vi "areaSettiingDlg.vi"(8 "error in (no error)":errorcluster caption="错误输入（无错误）", 11 "区域管理":T1 {"电极排列方式" items=["等间隔十字排列", "等间隔一字排列", "等间隔错位排列"]}) -> (0 "error out":errorcluster caption="错误输出（无错误）", 3 "区域管理 out":T1)   [LabVIEW 2014, in "SettingD.lvlib"]
uses:
  SettingD.llb/SettingD.lvlib
  DataBase/DataBase.lvlib
panel:
  in  "OK":bool
  in  "取消按钮":bool
  in  "确定按钮":bool
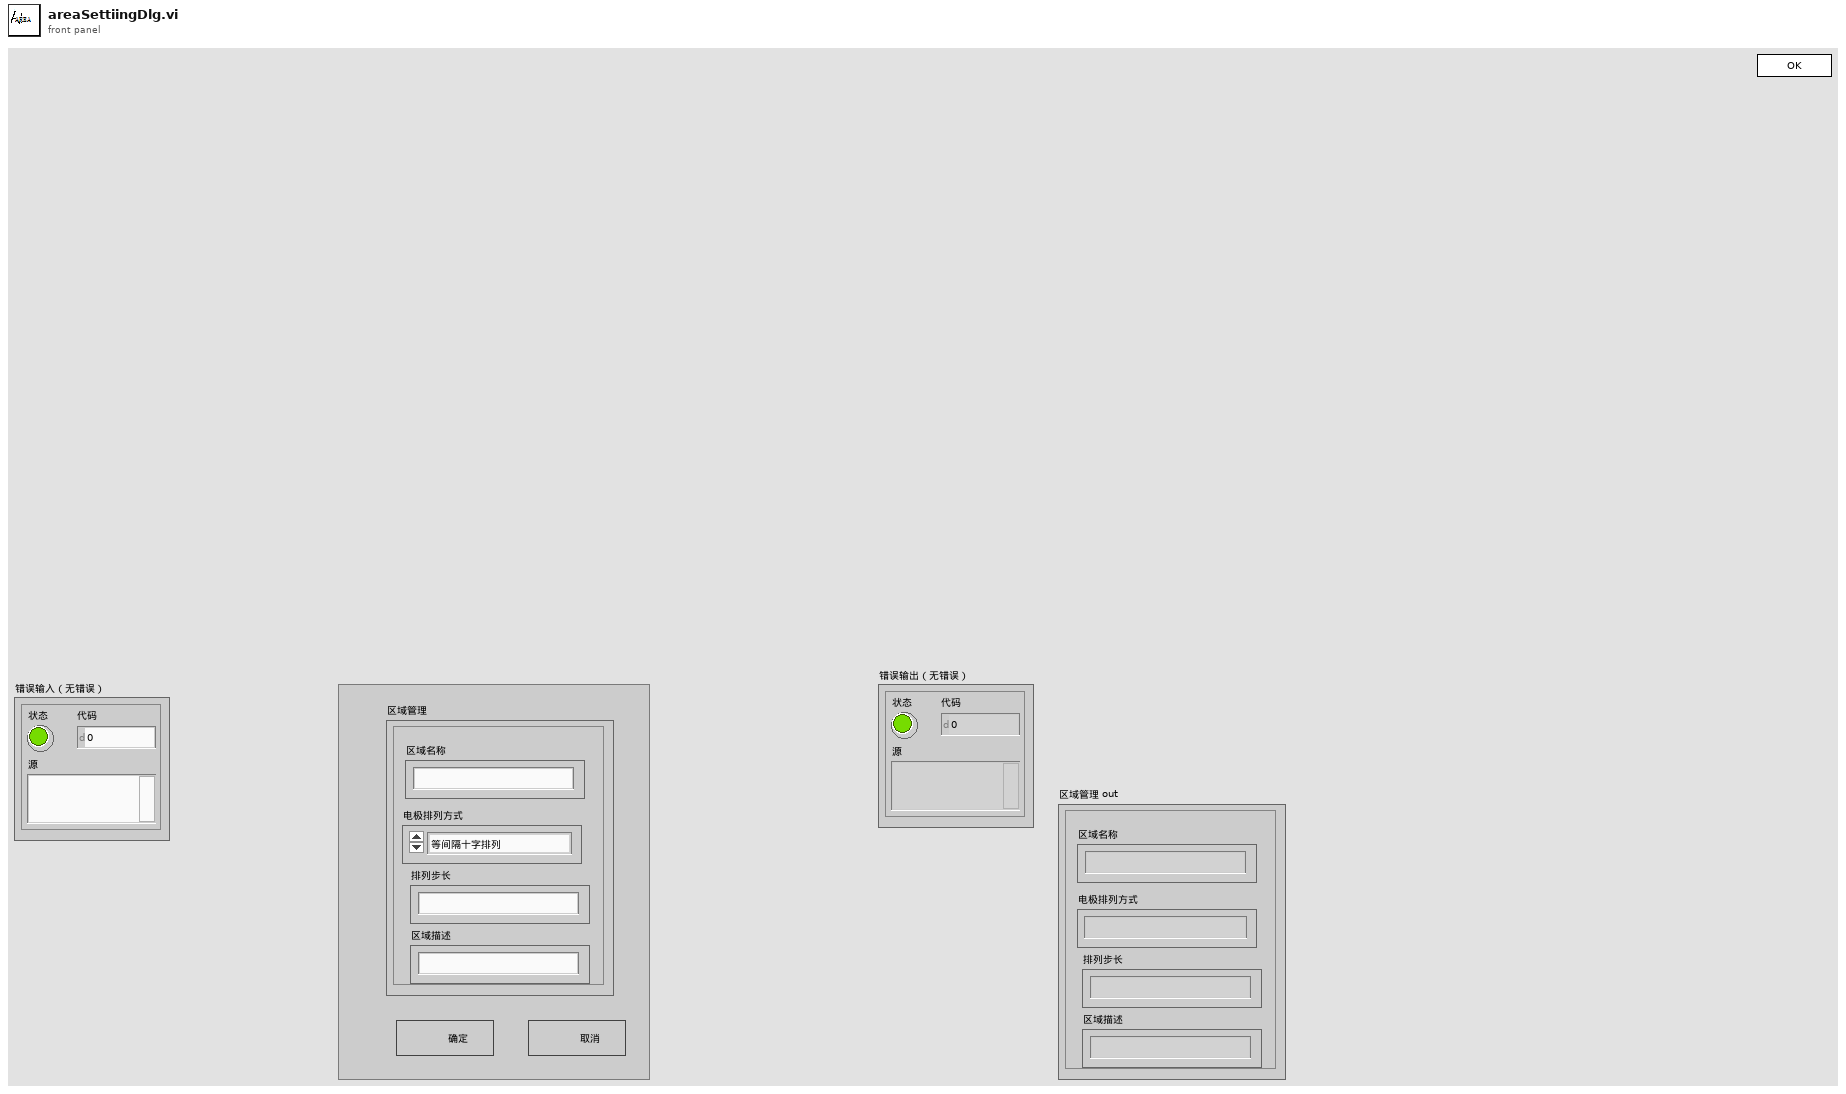
[diagram p1: front panel]
types:
  T1 = cluster{"区域名称":string, "电极排列方式":u16, "排列步长":string, "区域描述":string}
  T2 = enum32{"invalid app kind", "Development System", "Run Time System", "Student Edition", "Embedded LabVIEW", "Evaluation", "Custom"}
  T3 = enum32{"Invalid", "Standard", "Closed", "Hidden", "Minimized", "Maximized"}
  T4 = cluster{i32, "区域名称":string, string, "排列步长":string, "区域描述":string}
  T5 = cluster{"Core":cluster{"Current VI Reference":refnum<vi>, "Close Panel on Exit?":bool}, "Your Boolean data":bool, "Your string data":string}
  T6 = cluster{"Current VI Reference":refnum<vi>, "Close Panel on Exit?":bool}
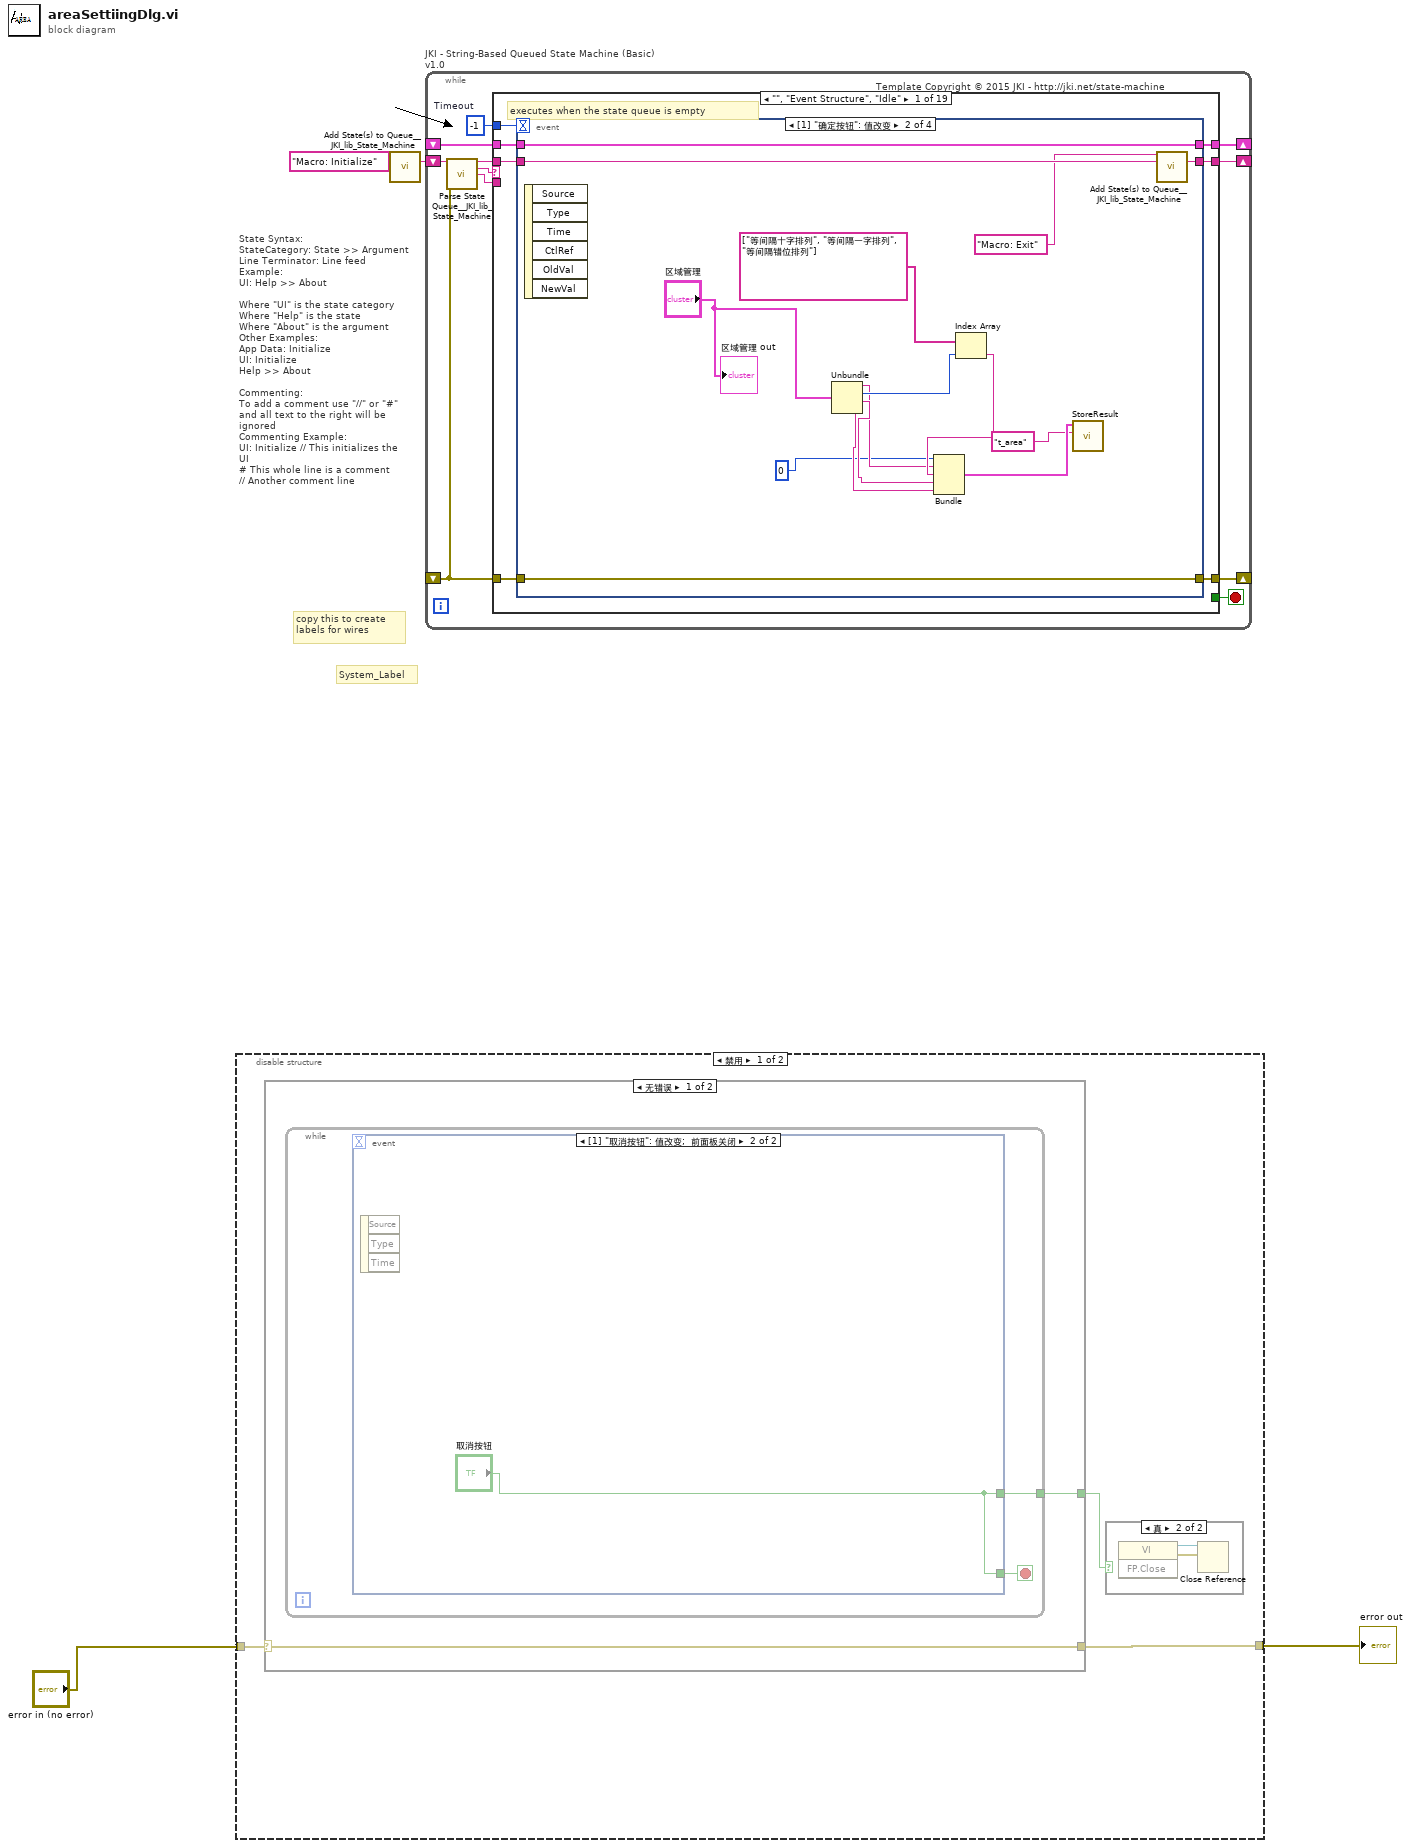
[diagram p0: block diagram]
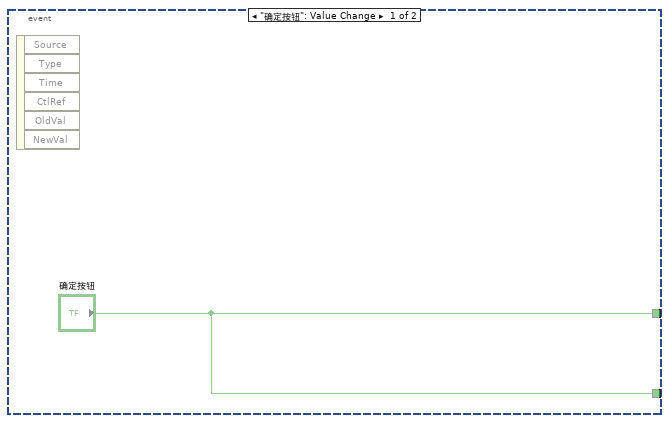
[diagram p2: hidden frame]
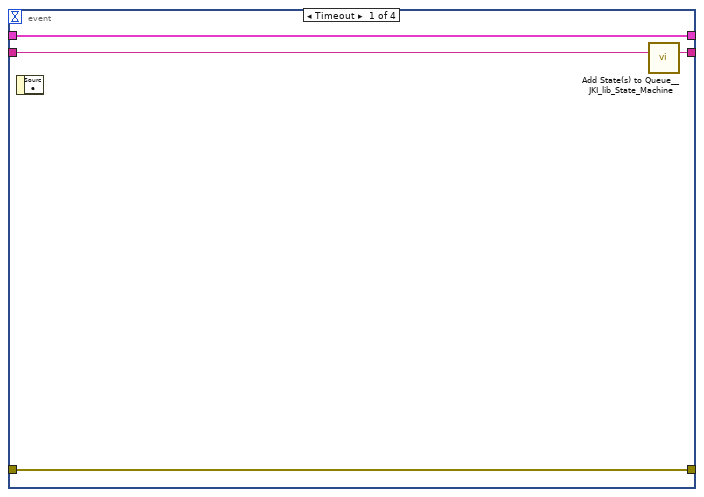
[diagram p6: hidden frame]
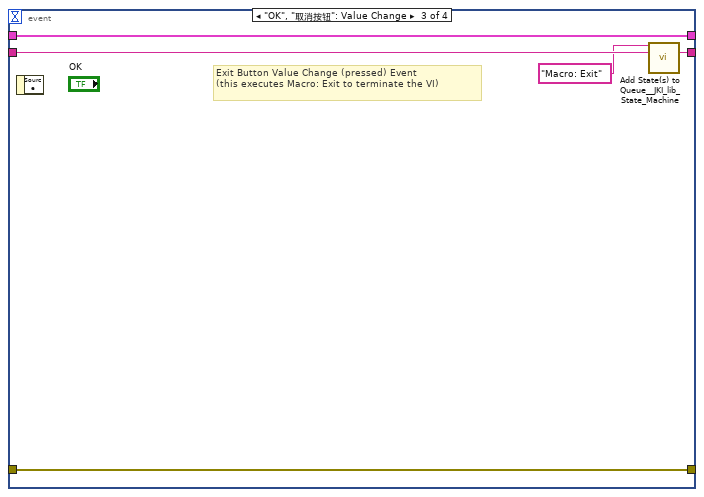
[diagram p7: hidden frame]
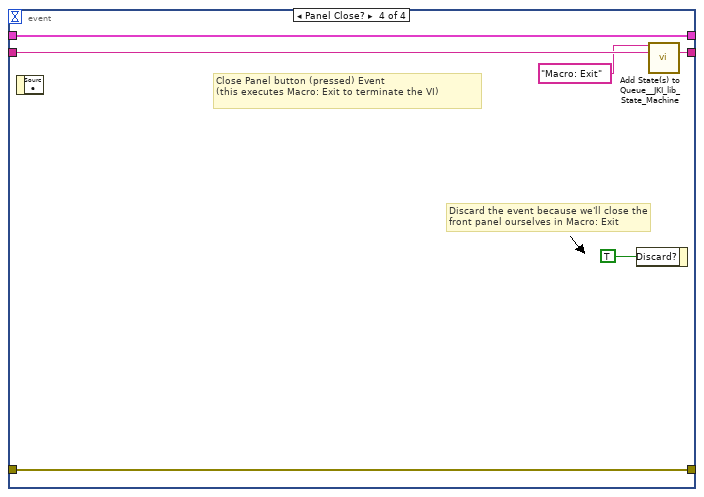
[diagram p8: hidden frame]
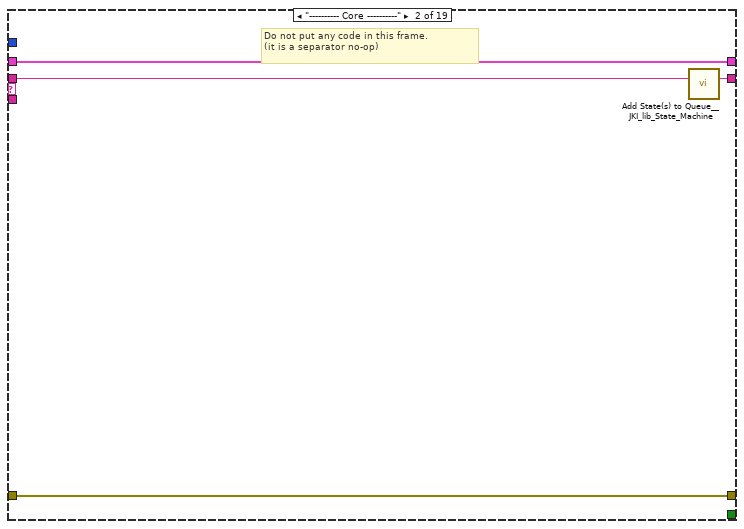
[diagram p9: hidden frame]
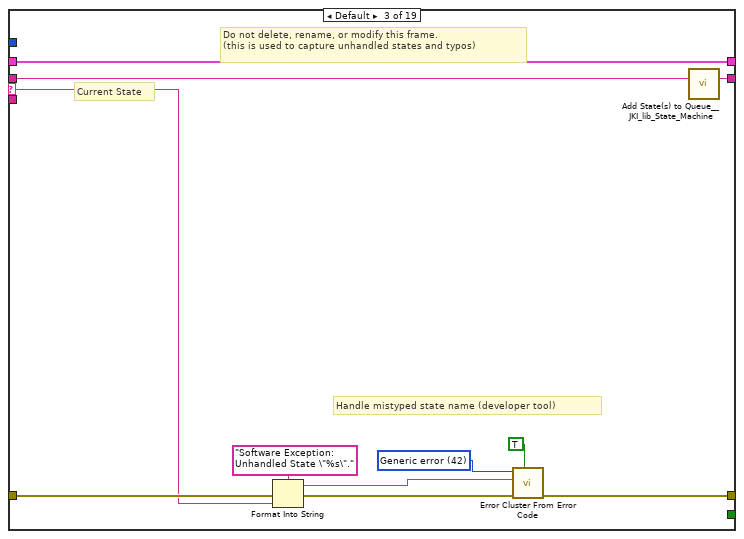
[diagram p10: hidden frame]
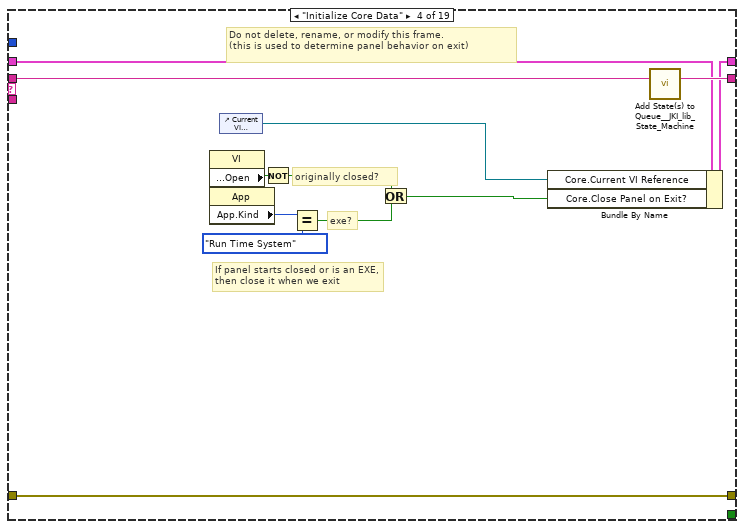
[diagram p11: hidden frame]
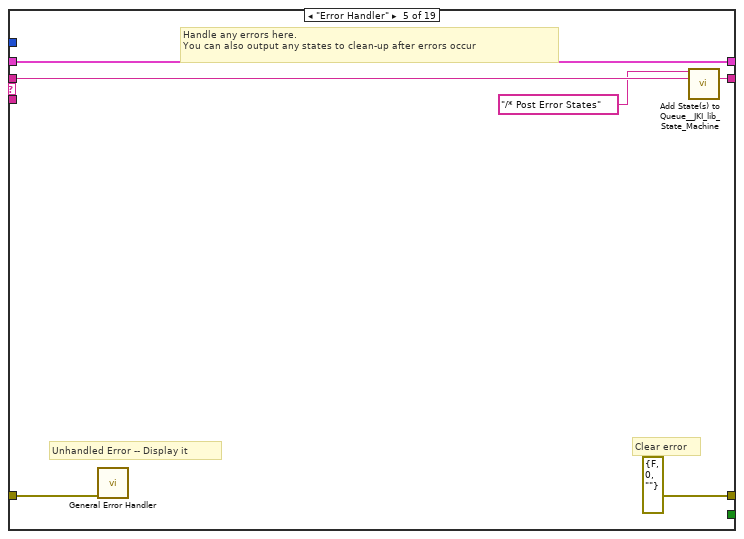
[diagram p12: hidden frame]
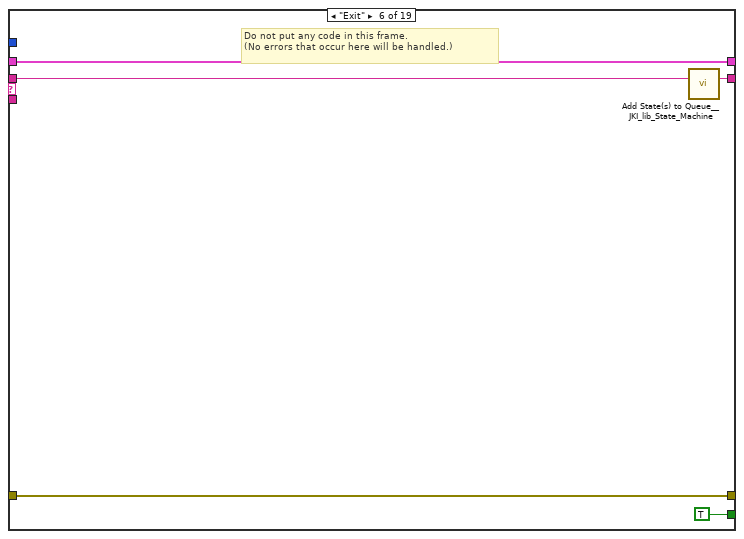
[diagram p13: hidden frame]
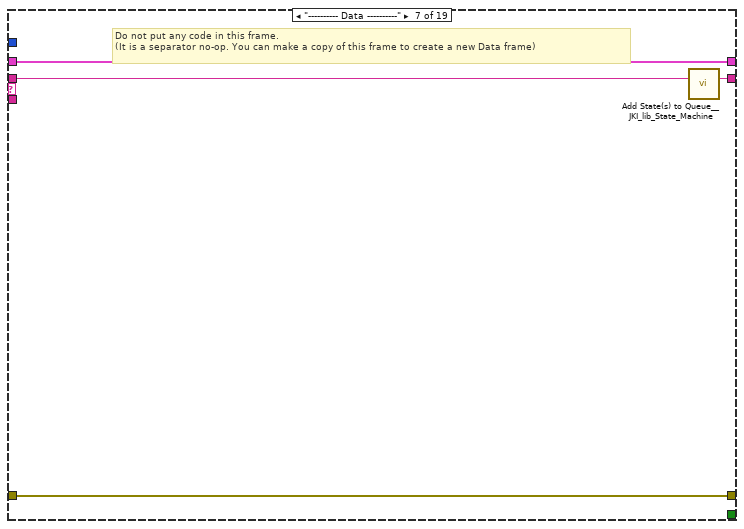
[diagram p14: hidden frame]
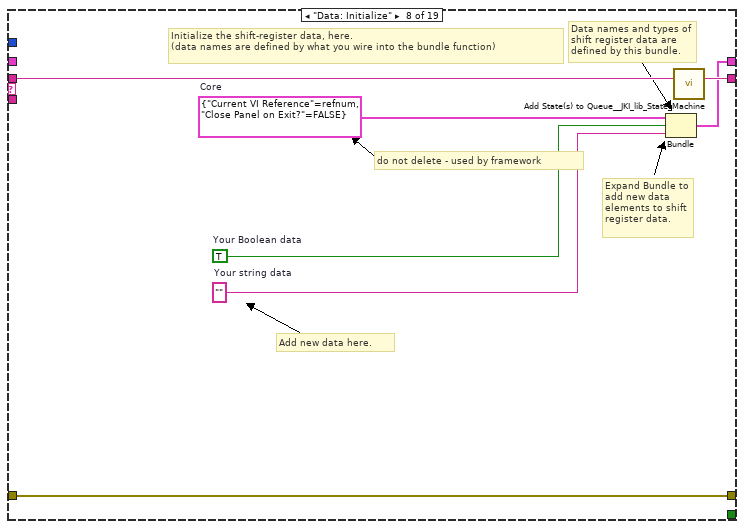
[diagram p15: hidden frame]
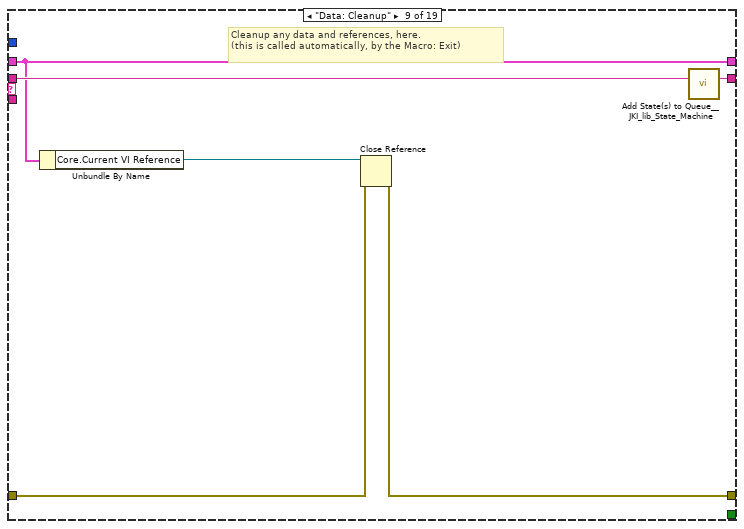
[diagram p16: hidden frame]
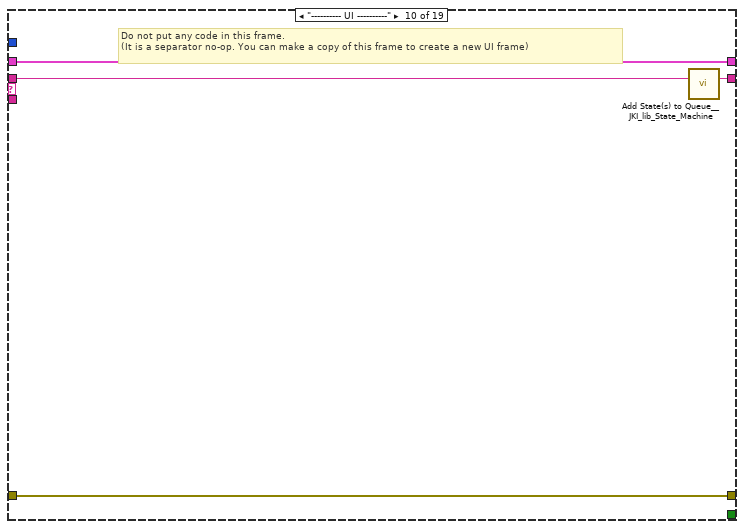
[diagram p17: hidden frame]
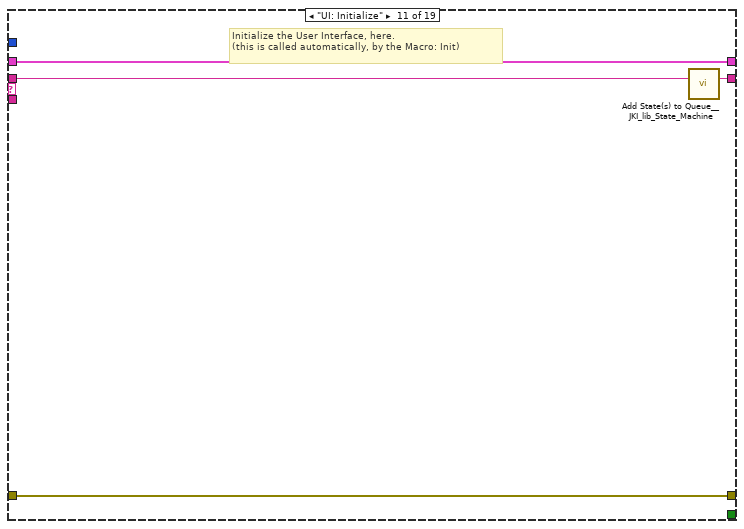
[diagram p18: hidden frame]
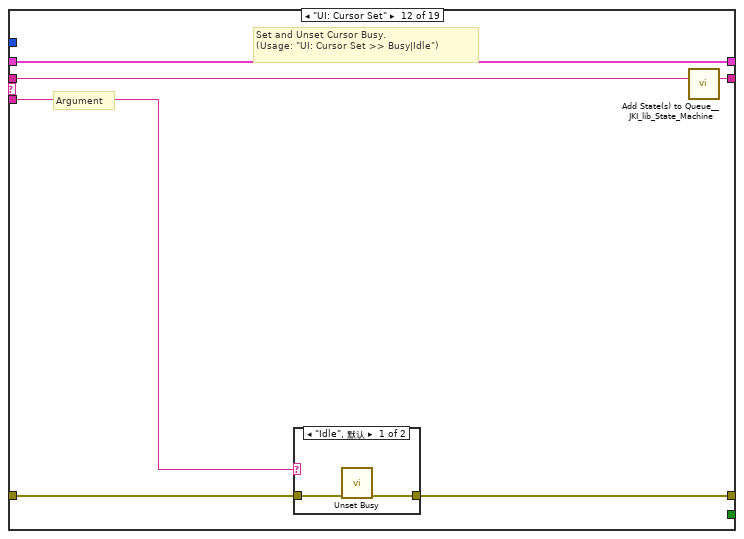
[diagram p19: hidden frame]
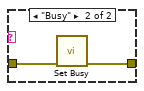
[diagram p20: hidden frame]
diagram:
  # "State Syntax:\nStateCategory: State >> Argument\nLine Terminator: Line feed\nExample:\nUI: Help >> About\n\nWhere \"UI\" is the state category\nWhere \"Help\" is the state\nWhere \"About\" is the argument\nOther Examples:\nApp Data: Initialize\nUI: Initialize\nHelp >> About\n\nCommenting:\nTo add a comment use \"//\" or \"#\" and all text to the right will be ignored\nCommenting Example:\nUI: Initialize // This initializes the UI\n# This whole line is a comment\n// Another comment line"
  # "copy this to create labels for wires"
  # "System_Label"
  n1 = disable-structure shown="禁用" {
    disable-tunnel: "error in (no error)" -> [w7 _]
    disable-tunnel: [w6 _] -> w3
    frame Disabled {
      n2 = case shown="无错误" w7 {
        selector: w7 -> [w9 w14]
        tunnel: [w9 w14] -> w6
        tunnel: [w8 _] -> w5
        frame No Error {
          n3 = while {
            tunnel: [w11] -> w8
            stop <- w10 stop-if-true
            n4 = event shown="[1] \"取消按钮\": 值改变;  前面板关闭" {
              selector: _ -> [_ _]
              dyn-events: _ -> [_ _]
              timeout: _ -> [_ _]
              tunnel: ["确定按钮" "取消按钮"] -> w11
              tunnel: ["确定按钮" "取消按钮"] -> w10
              event "确定按钮": Value Change {
                n5 = event-data() -> ()  [unwired: 1 in, 6 out]
              }
              event "取消按钮": Value Change; Panel Close {
                n6 = event-data() -> ()  [unwired: 1 in, 3 out]
              }
            }
          }
        }
        frame Error {
        }
      }
      n7 = case shown="真" w5 {
        frame False {
        }
        frame True {
          n8 = invoke class="VI" method="FP.Close"() -> (reference out=w16:refnum<vi>, error out=w15:errorcluster)  [unwired: 3 in, 1 out]
          n9 = Close Reference(reference=w16, error in (no error)=w15) -> ()  [unwired: 1 out]
        }
      }
    }
    frame Enabled {
    }
  }
  "error out" <- w3
  n10 = call <vilib>:"Add State(s) to Queue__JKI_lib_State_Machine.vi"("State(s) in (\"\")"="Macro: Initialize") -> ("States Out"=w2:string)  [unwired: 14 in]
  n11 = while "JKI - String-Based Queued State Machine (Basic) v1.0" {
    shift-right: [w20] -> _
    shift-left: _ -> [w19]
    shift-right: [w23] -> _
    shift-left: _ -> [w17]
    shift-right: [w22] -> _
    shift-left: w2 -> [w24]
    stop <- w21 stop-if-true
    w18 = -1  # Timeout
    # "Template Copyright © 2015 JKI - http://jki.net/state-machine"
    n12 = call <vilib>:"Parse State Queue__JKI_lib_State_Machine.vi"("State Queue"=w24, "Error In (no error)"=w17) -> ("Remaining States"=w26:string, "Current State"=w27:string, "Arguments"=w25:string)  [unwired: 11 in]
    n13 = case shown="\"\", \"Event Structure\", \"Idle\"" w27 {
      selector: w27 -> [_ _ w69 _ _ _ _ _ _ _ _ _ _ _ _ _ _ _ _]
      tunnel: w26 -> [w34 w68 w73 w91 w97 w102 w106 w113 w119 w123 w127 w133 w144 w170 w175 w185 w189 w193 w197]
      tunnel: w25 -> [_ _ _ _ _ _ _ _ _ _ _ w128 w138 _ _ _ _ _ _]
      tunnel: w19 -> [w32 w65 w71 w82 w94 w100 w103 _ w114 w120 w125 w131 w140 w167 w172 w182 w186 w190 w194]
      tunnel: [w31 w66 w75 w88 errorcluster {"status"=FALSE, "code"=0, "source"=""} ("error out") w99 w104 w110 w115 w121 w124 w129 w141 w168 w173 w183 w187 w191 w195] -> w23
      tunnel: w17 -> [w30 w66 w74 w88 w93 w99 w104 w110 w116 w121 w124 w130 w142 w168 w173 w183 w187 w191 w195]
      tunnel: [w33 w67 w72 w90 w96 w101 w105 w112 w118 w122 w126 w132 w143 w169 w174 w184 w188 w192 w196] -> w22
      tunnel: [_ _ _ _ _ TRUE _ _ _ _ _ _ _ _ _ _ _ _ _] -> w21
      tunnel: [w29 w65 w71 w89 w94 w100 w103 w111 w114 w120 w125 w131 w140 w167 w172 w182 w186 w190 w194] -> w20
      tunnel: w18 -> [w28 _ _ _ _ _ _ _ _ _ _ _ _ _ _ _ _ _ _]
      frame "", "Event Structure", "Idle" {
        # "executes when the state queue is empty"
        n14 = event shown="[1] \"确定按钮\": 值改变" {
          selector: _ -> [_ _ _ _]
          dyn-events: _ -> [_ _ _ _]
          timeout: w28 -> [_ _ _ _]
          tunnel: w34 -> [w38 w53 w58 w64]
          tunnel: [w37 w52 w57 w63] -> w33
          tunnel: w32 -> [w35 w50 w55 w61]
          tunnel: [w36 w51 w56 w62] -> w31
          tunnel: w30 -> [w36 w51 w56 w62]
          tunnel: [w35 w50 w55 w61] -> w29
          event Timeout {
            n15 = event-data() -> ()  [unwired: 1 in, 1 out]
            n16 = call <vilib>:"Add State(s) to Queue__JKI_lib_State_Machine.vi"("State(s) in (\"\")"=w38) -> ("States Out"=w37:string)  [unwired: 14 in]
          }
          event "确定按钮": Value Change {
            n17 = event-data() -> ()  [unwired: 1 in, 6 out]
            n18 = Unbundle("区域管理") -> ("区域名称"=w43:string, "电极排列方式"=w47:u16, "排列步长"=w44:string, "区域描述"=w45:string)
            n19 = Index Array(array=string[] ["等间隔十字排列", "等间隔一字排列", "等间隔错位排列"], index=w47) -> (element=w48:string)
            n20 = Bundle(0, "区域名称"=w43, w48, "排列步长"=w44, "区域描述"=w45) -> (w49:T4)  [unwired: 1 in]
            n21 = call "StoreResult.vi"("Table name"="t_area", "区域管理"=w49) -> ()  [unwired: 9 in, 1 out]
            n22 = call <vilib>:"Add State(s) to Queue__JKI_lib_State_Machine.vi"("State(s) in Front (\"\")"="Macro: Exit", "State(s) in (\"\")"=w53) -> ("States Out"=w52:string)  [unwired: 13 in]
            "区域管理 out" <- "区域管理"
          }
          event "OK", "取消按钮": Value Change {
            # "Exit Button Value Change (pressed) Event\n(this executes Macro: Exit to terminate the VI)"
            n23 = event-data() -> ()  [unwired: 1 in, 1 out]
            n24 = call <vilib>:"Add State(s) to Queue__JKI_lib_State_Machine.vi"("State(s) in Front (\"\")"="Macro: Exit", "State(s) in (\"\")"=w58) -> ("States Out"=w57:string)  [unwired: 13 in]
          }
          event Panel Close? {
            # "Discard the event because we'll close the front panel ourselves in Macro: Exit"
            # "Close Panel button (pressed) Event\n(this executes Macro: Exit to terminate the VI)"
            n25 = event-data() -> ()  [unwired: 1 in, 1 out]
            n26 = event-data("Discard?"=TRUE) -> ()  [unwired: 1 in, 1 out]
            n27 = call <vilib>:"Add State(s) to Queue__JKI_lib_State_Machine.vi"("State(s) in Front (\"\")"="Macro: Exit", "State(s) in (\"\")"=w64) -> ("States Out"=w63:string)  [unwired: 13 in]
          }
        }
      }
      frame "---------- Core ----------" {
        # "Do not put any code in this frame.\n(it is a separator no-op)"
        n28 = call <vilib>:"Add State(s) to Queue__JKI_lib_State_Machine.vi"("State(s) in (\"\")"=w68) -> ("States Out"=w67:string)  [unwired: 14 in]
      }
      frame Default {
        w78 = 42 items=["No error", "Argument error", "Memory is full", "Out of zone", "End of file", "File already open", "Generic file I/O error", "File not found", "File permission error", "Disk is full", "Duplicate path", "Too many files open", "System feature not enabled", "Resource file not found", "Cannot add resource", "Resource not found", "Image not found", "Image memory error", "Pen does not exist", "Config type invalid", "Config token not found", "Config parse error", "Config memory error", "Bad external code format", "Bad external code offset", "External code not present", "Null window", "Destroy window error", "Null menu", "Print aborted", "Bad print record", "Print driver error", "Windows error during printing", "Memory error during printing", "Print dialog error", "Generic print error", "Invalid device refnum", "Device not found", "Device parameter error", "Device unit error", "Cannot open device", "Device call aborted", "Generic error", "Cancelled by user", "Object ID too low", "Object ID too high", "Object not in heap", "Unknown heap", "Unknown object (invalid DefProc)", "Unknown object (DefProc not in table)", "Message out of range", "Invalid (null) method", "Unknown message", "Manager call not supported", "Bad address", "Network operation in progress", "Network operation timed out", "Connection is busy", "Network attribute not supported", "Network error", "Address in use", "System out of memory", "Connection aborted", "Connection refused", "Not connected", "Already connected", "Connection closed", "Initialization error (interapplication manager)", "Bad occurrence", "Wait on unbound occurrence handler", "Occurrence queue overflow", "Datalog type conflict", "Unused", "Unrecognized type (interapplication manager)", "Memory corrupt", "Failed to make temporary DLL", "Old CIN version", "Drag socket not found", "Failed to load drop-object", "Failed to register OLE object", "Failed to release OLE object", "Format specifier type mismatch", "Unknown format specifier", "Too few format specifiers", "Too many format specifiers", "Scan failed", "Newer CIN version", "Error converting to variant", "Runtime menu error", "Password tampered", "Variant attribute not found", "Incompatible variant data type", "Event data is not available", "Event Store is not present", "Occurrence is not found", "Event Queue is not created", "Event info is not available", "Refnum passed is NULL", "Error retrieving Class GUID", "Error retrieving CoClass GUID", "Error retrieving TypeLib GUID.", "Bad built application magic bytes.", "Specific driver is different from the specific driver associated with the Logical Name.", "There is no session opened to the class driver.", "Max Error", "MAX - Error with config objects", "MAX - Error loading configuration", "MAX - Group not supported"]
        # "Current State"
        # "Do not delete, rename, or modify this frame.\n(this is used to capture unhandled states and typos)"
        # "Handle mistyped state name (developer tool)"
        n29 = Format Into String(format string="Software Exception: Unhandled State \"%s\"." ("message"), error in=w74, w69) -> (resulting string=w77:string, error out=w76:errorcluster)  [unwired: 1 in]
        n30 = call <vilib>:"Error Cluster From Error Code.vi"("show call chain? (False)"=TRUE, "error in (no error)"=w76, "error message (\"\")"=w77, "error code (0)"=w78) -> ("error out"=w75:errorcluster)  [unwired: 5 in]
        n31 = call <vilib>:"Add State(s) to Queue__JKI_lib_State_Machine.vi"("State(s) in (\"\")"=w73) -> ("States Out"=w72:string)  [unwired: 14 in]
      }
      frame "Initialize Core Data" {
        # "Do not delete, rename, or modify this frame.\n(this is used to determine panel behavior on exit)"
        # "originally closed?"
        # "exe?"
        # "If panel starts closed or is an EXE, then close it when we exit"
        n32 = property class="VI"() -> ("Front Panel.Open"=w87:bool)  [unwired: 2 in, 2 out]
        n33 = property class="App"() -> ("App.Kind"=w86:T2)  [unwired: 2 in, 2 out]
        n34 = control-ref of="Current VI Reference"() -> (w80:refnum<vi>)
        n35 = Not(x=w87) -> (.not. x?=w84:bool)
        n36 = Equal?(x=w86, y=T2."Run Time System" ("Application:Kind")) -> (x = y?=w83:bool)
        n37 = Or(x=w84, y=w83) -> (x .or. y?=w81:bool)
        n38 = Bundle By Name(cluster=w82, "Core.Current VI Reference"=w80, "Core.Close Panel on Exit?"=w81) -> (w89:T5)
        n39 = call <vilib>:"Add State(s) to Queue__JKI_lib_State_Machine.vi"("State(s) in (\"\")"=w91) -> ("States Out"=w90:string)  [unwired: 14 in]
      }
      frame "Error Handler" {
        # "Unhandled Error -- Display it"
        # "Handle any errors here.\nYou can also output any states to clean-up after errors occur"
        # "Clear error"
        n40 = call <vilib>:"General Error Handler.vi"("error in (no error)"=w93) -> ()  [unwired: 10 in, 5 out]
        n41 = call <vilib>:"Add State(s) to Queue__JKI_lib_State_Machine.vi"("State(s) in Front (\"\")"="/* Post Error States", "State(s) in (\"\")"=w97) -> ("States Out"=w96:string)  [unwired: 13 in]
      }
      frame "Exit" {
        # "Do not put any code in this frame.\n(No errors that occur here will be handled.)"
        n42 = call <vilib>:"Add State(s) to Queue__JKI_lib_State_Machine.vi"("State(s) in (\"\")"=w102) -> ("States Out"=w101:string)  [unwired: 14 in]
      }
      frame "---------- Data ----------" {
        # "Do not put any code in this frame.\n(It is a separator no-op. You can make a copy of this frame to create a new Data frame)"
        n43 = call <vilib>:"Add State(s) to Queue__JKI_lib_State_Machine.vi"("State(s) in (\"\")"=w106) -> ("States Out"=w105:string)  [unwired: 14 in]
      }
      frame "Data: Initialize" {
        w107 = T6 {"Current VI Reference"=refnum, "Close Panel on Exit?"=FALSE}  # Core
        w109 = TRUE  # Your Boolean data
        w108 = ""  # Your string data
        # "do not delete - used by framework"
        # "Expand Bundle to add new data elements to shift register data."
        # "Add new data here."
        # "Data names and types of shift register data are defined by this bundle."
        # "Initialize the shift-register data, here.\n(data names are defined by what you wire into the bundle function)"
        n44 = Bundle("Core"=w107, "Your Boolean data"=w109, "Your string data"=w108) -> (w111:T5)  [unwired: 1 in]
        n45 = call <vilib>:"Add State(s) to Queue__JKI_lib_State_Machine.vi"("State(s) in (\"\")"=w113) -> ("States Out"=w112:string)  [unwired: 14 in]
      }
      frame "Data: Cleanup" {
        # "Cleanup any data and references, here.\n(this is called automatically, by the Macro: Exit)"
        n46 = Unbundle By Name(w114) -> ("Core.Current VI Reference"=w117:refnum<vi>)
        n47 = Close Reference(reference=w117, error in (no error)=w116) -> (error out=w115:errorcluster)
        n48 = call <vilib>:"Add State(s) to Queue__JKI_lib_State_Machine.vi"("State(s) in (\"\")"=w119) -> ("States Out"=w118:string)  [unwired: 14 in]
      }
      frame "---------- UI ----------" {
        # "Do not put any code in this frame.\n(It is a separator no-op. You can make a copy of this frame to create a new UI frame)"
        n49 = call <vilib>:"Add State(s) to Queue__JKI_lib_State_Machine.vi"("State(s) in (\"\")"=w123) -> ("States Out"=w122:string)  [unwired: 14 in]
      }
      frame "UI: Initialize" {
        # "Initialize the User Interface, here.\n(this is called automatically, by the Macro: Init)"
        n50 = call <vilib>:"Add State(s) to Queue__JKI_lib_State_Machine.vi"("State(s) in (\"\")"=w127) -> ("States Out"=w126:string)  [unwired: 14 in]
      }
      frame "UI: Cursor Set" {
        # "Argument"
        # "Set and Unset Cursor Busy.\n(Usage: \"UI: Cursor Set >> Busy|Idle\")"
        n51 = case shown="\"Idle\", 默认" w128 {
          tunnel: w130 -> [w135 w137]
          tunnel: [w134 w136] -> w129
          frame "Idle", Default {
            n52 = call <vilib>:"Unset Busy.vi"("error in (no error)"=w135) -> ("error out"=w134:errorcluster)  [unwired: 10 in]
          }
          frame "Busy" {
            n53 = call <vilib>:"Set Busy.vi"("error in (no error)"=w137) -> ("error out"=w136:errorcluster)  [unwired: 9 in, 1 out]
          }
        }
        n54 = call <vilib>:"Add State(s) to Queue__JKI_lib_State_Machine.vi"("State(s) in (\"\")"=w133) -> ("States Out"=w132:string)  [unwired: 14 in]
      }
      frame "UI: Front Panel State" {
        # "Argument"
        # "Set Front Panel Open or Closed\n(Usage: \"UI: Front Panel State >> Open|Close\")"
        n55 = Unbundle By Name(w140) -> ("Core.Current VI Reference"=w139:refnum<vi>)
        n56 = case shown="\"Open\", 默认" w138 {
          tunnel: w142 -> [w148 w161]
          tunnel: [w150 w162] -> w141
          tunnel: w139 -> [w149 w159]
          frame "Open", Default {
            n57 = property class="VI"(reference=w149, error in=w148) -> (reference out=w146:refnum<vi>, error out=w147:errorcluster, "Front Panel.Open"=w145:bool)
            n58 = case shown="假" w145 {
              tunnel: [w153 w156] -> w150
              tunnel: w147 -> [w152 w156]
              tunnel: w146 -> [w151 _]
              frame False {
                n59 = invoke class="VI" method="FP.Open"(reference=w151, error in=w152, "Activate"=TRUE, "State"=T3."Standard") -> (error out=w153:errorcluster)  [unwired: 1 in, 4 out]
              }
              frame True {
              }
            }
          }
          frame "Close" {
            n60 = property class="VI"(reference=w159, error in=w161) -> (reference out=w158:refnum<vi>, error out=w160:errorcluster, "Front Panel.Open"=w157:bool)
            n61 = case shown="真" w157 {
              tunnel: [w163 w166] -> w162
              tunnel: w160 -> [w163 w165]
              tunnel: w158 -> [_ w164]
              frame False {
              }
              frame True {
                n62 = invoke class="VI" method="FP.Close"(reference=w164, error in=w165) -> (error out=w166:errorcluster)  [unwired: 1 in, 2 out]
              }
            }
          }
        }
        n63 = call <vilib>:"Add State(s) to Queue__JKI_lib_State_Machine.vi"("State(s) in (\"\")"=w144) -> ("States Out"=w143:string)  [unwired: 14 in]
      }
      frame "---------- Macro ----------" {
        # "Do not put any code in this frame.\n(It is a separator no-op. You can make a copy of this frame to create a new Macro frame)"
        n64 = call <vilib>:"Add State(s) to Queue__JKI_lib_State_Machine.vi"("State(s) in (\"\")"=w170) -> ("States Out"=w169:string)  [unwired: 14 in]
      }
      frame "Macro: Initialize" {
        w171 = "Data: Initialize\nInitialize Core Data\nUI: Initialize\nUI: Front Panel State >> Open"  # Data: Initialize Initialize Core Data UI: Initialize UI: Front Panel State >> Open
        # "Initialization Macro\n(This is called once, when the VI starts)"
        n65 = call <vilib>:"Add State(s) to Queue__JKI_lib_State_Machine.vi"("State(s) in Front (\"\")"=w171, "State(s) in (\"\")"=w175) -> ("States Out"=w174:string)  [unwired: 13 in]
      }
      frame "Macro: Exit" {
        # "Exit Macro\n(This is called once, when the VI exits)"
        n66 = Unbundle By Name(w182) -> ("Core.Close Panel on Exit?"=w181:bool)
        n67 = Select(t="UI: Front Panel State >> Close", s=w181, f="") -> (s? t:f=w178:string)
        n68 = call <vilib>:"Add State(s) to Queue__JKI_lib_State_Machine.vi"("State(s) in (\"\")"=w178, "State(s) at Back (\"\")"="Data: Cleanup\nExit") -> ("States Out"=w176:string)  [unwired: 13 in]
        n69 = call <vilib>:"Add State(s) to Queue__JKI_lib_State_Machine.vi"("State(s) in Front (\"\")"=w176, "State(s) in (\"\")"=w185) -> ("States Out"=w184:string)  [unwired: 13 in]
      }
      frame "---------- New Category ----------" {
        # "Template Separator\n(You can make a copy of, or modify, this frame)"
        n70 = call <vilib>:"Add State(s) to Queue__JKI_lib_State_Machine.vi"("State(s) in (\"\")"=w189) -> ("States Out"=w188:string)  [unwired: 14 in]
      }
      frame "New Category: 1" {
        # "Your code here.\n(You can make a copy of, or modify, this frame)"
        n71 = call <vilib>:"Add State(s) to Queue__JKI_lib_State_Machine.vi"("State(s) in (\"\")"=w193) -> ("States Out"=w192:string)  [unwired: 14 in]
      }
      frame "New Category: 2" {
        # "Your code here.\n(You can make a copy of, or modify, this frame)"
        n72 = call <vilib>:"Add State(s) to Queue__JKI_lib_State_Machine.vi"("State(s) in (\"\")"=w197) -> ("States Out"=w196:string)  [unwired: 14 in]
      }
    }
  }
